vi "Get_Arguments.vi"(8 "error in (no error)":errorcluster caption="entrée d'erreur (pas d'erreur)", 11 "Process (Default) en entrée":refnum<class "Process (Default).lvclass">) -> (0 "error out":errorcluster caption="sortie d'erreur", 2 "Arguments":string, 3 "Process (Default) en sortie":refnum<class "Process (Default).lvclass">)   [LabVIEW 2020, in "Library Instrument & Equipement.lvlib" / "Process (Default).lvclass"]
uses:
  Process (Default).lvclass
  Process (Default).lvclass/Process (Default).ctl
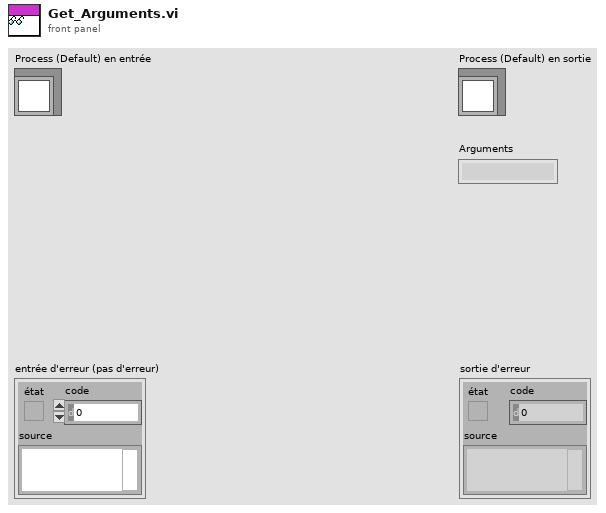
[diagram p1: front panel]
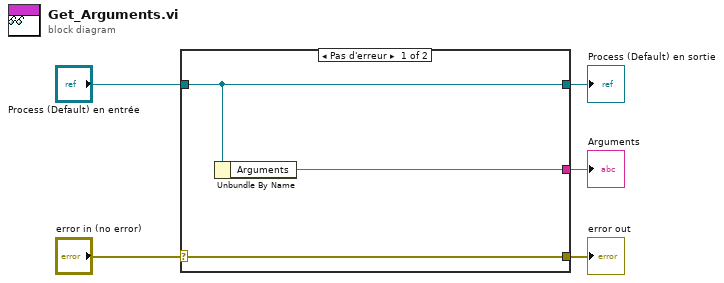
[diagram p0: block diagram]
diagram:
  n1 = case shown="Pas d'erreur" "error in (no error)" {
    selector: "error in (no error)" -> [w8 w9]
    tunnel: [w8 w9] -> w4
    tunnel: [w7 w10] -> w2
    tunnel: "Process (Default) en entrée" -> [w7 w10]
    tunnel: [w6 _] -> w1
    frame No Error {
      n2 = Unbundle By Name(w7) -> ("Arguments"=w6:string)
    }
    frame Error {
    }
  }
  "error out" <- w4
  "Process (Default) en sortie" <- w2
  "Arguments" <- w1
